vi "Equi-Ripple BandStop PtByPt.vi"(0 "x":dbl format="%0.2f", 1 "lower pass freq":dbl=0.125 format="%0.2f", 2 "higher pass freq":dbl=0.45 format="%0.2f", 3 "initialize":bool, 7 "sampling freq: fs":dbl=1.0 format="%0.2f", 11 "# of taps":i32=31, 12 "lower stop freq":dbl=0.25000000000000006 format="%0.2f", 13 "higher stop freq":dbl=0.3500000000000001 format="%0.2f") -> (4 "Filtered x":dbl format="%0.2f", 15 "error":i32)   [LabVIEW 2017, in "NI_PtbyPt.lvlib"]
doc: "Filters <B>x</B> using an equi-ripple bandstop FIR filter model."
uses:
  <vilib>/ptbypt/NI_PtbyPt.lvlib
  <vilib>/Analysis/NI_AALBase.lvlib
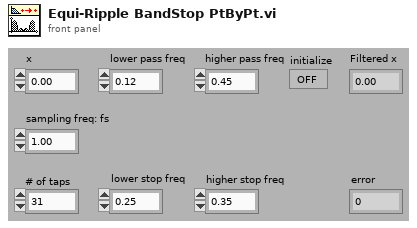
[diagram p1: front panel]
types:
  T1 = cluster{"Amplitude":dbl, "DC":dbl, "lower pass freq":dbl, "Weight":dbl}
  T2 = cluster{"Amplitude":dbl, "lower stop freq":dbl, "higher stop freq":dbl, "Weight":dbl}
  T3 = cluster{"Amplitude":dbl, "higher pass freq":dbl, dbl, "Weight":dbl}
  T4 = cluster{"Amplitude":dbl, "higher pass freq":dbl, "higher stop freq":dbl, "Weight":dbl}[]
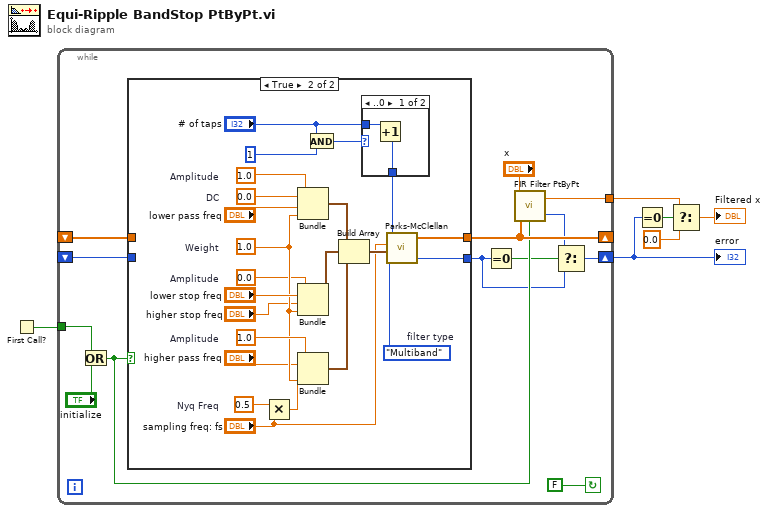
[diagram p0: block diagram]
diagram:
  n1 = First Call?() -> (First Call?: T/F=w6:bool)
  n2 = while {
    tunnel: w6 -> [w14]
    shift-left: _ -> [w17]
    shift-right: [w19] -> _
    shift-right: [w9] -> w5
    shift-left: _ -> [w8]
    tunnel: [w7] -> w3
    stop <- FALSE continue-if-true
    n3 = Or(x=w14, y="initialize") -> (x .or. y?=w15:bool)
    n4 = case shown="True" w15 {
      tunnel: [w21 w44] -> w19
      tunnel: w17 -> [w21 _]
      tunnel: [w20 w22] -> w10
      tunnel: w8 -> [w20 _]
      frame False {
      }
      frame True {
        w43 = 1.0  # Amplitude
        w42 = 0.0  # DC
        w33 = 1.0  # Weight
        w32 = 0.0  # Amplitude
        w36 = 0.5  # Nyq Freq
        w41 = 1.0  # Amplitude
        w25 = enum32{"Multiband", "Differentiator", "Hilbert"}."Multiband"  # filter type
        n5 = Multiply(x=w36, y="sampling freq: fs") -> (x*y=w29:dbl)
        n6 = Bundle("Amplitude"=w43, "DC"=w42, "lower pass freq"="lower pass freq", "Weight"=w33) -> (w37:T1)  [unwired: 1 out]
        n7 = Bundle("Amplitude"=w32, "lower stop freq"="lower stop freq", "higher stop freq"="higher stop freq", "Weight"=w33) -> (w28:T2)  [unwired: 1 out]
        n8 = Bundle("Amplitude"=w41, "higher pass freq"="higher pass freq", w29, "Weight"=w33) -> (w40:T3)  [unwired: 1 out]
        n9 = And(x="# of taps", y=1) -> (x .and. y?=w39:i32)
        n10 = Build Array(w37, w28, w40) -> (w27:T4)
        n11 = case shown="..0" w39 {
          tunnel: [w46 w47] -> w23
          tunnel: "# of taps" -> [w45 w47]
          frame ..0 {
            n12 = Increment(x=w45) -> (x+1=w46:i32)
          }
          frame 1.. {
          }
        }
        n13 = call <vilib>:"Parks-McClellan.vi"("filter type"=w25, "Band Parameters"=w27, "sampling freq: fs"="sampling freq: fs", "# of taps"=w23) -> ("error"=w22:i32, "h"=w44:dbl[])  [unwired: 1 out]
      }
    }
    n14 = Equal To 0?(x=w10) -> (x = 0?=w12:bool)
    n15 = call <vilib>:"FIR Filter PtByPt.vi"("initialize"=w15, "Forward Coefficients"=w19, "x"="x") -> ("error"=w11:i32, "Filtered x"=w7:dbl)  [unwired: 1 out]
    n16 = Select(t=w11, s=w12, f=w10) -> (s? t:f=w9:i32)
  }
  "error" <- w5
  n17 = Equal To 0?(x=w5) -> (x = 0?=w4:bool)
  n18 = Select(t=w3, s=w4, f=0.0) -> (s? t:f=→"Filtered x":dbl)
